vi "Generate a random block.vi"() -> (1 "Block Array":u8[][](array[numeric]))   [LabVIEW 2019]
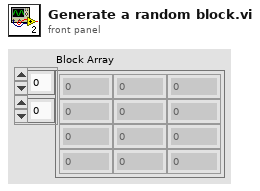
[diagram p1: front panel]
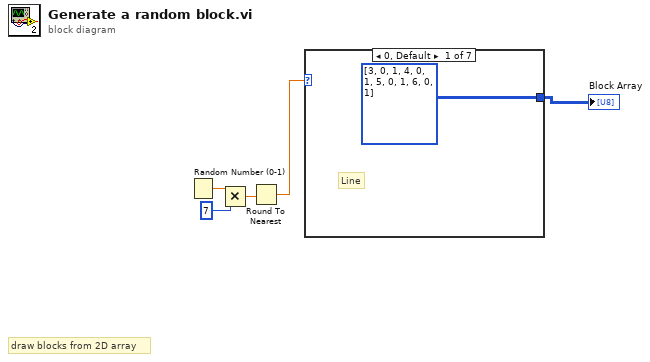
[diagram p0: block diagram]
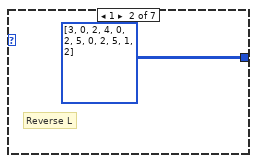
[diagram p2: hidden frame]
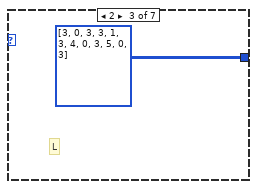
[diagram p3: hidden frame]
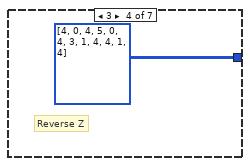
[diagram p4: hidden frame]
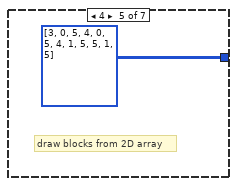
[diagram p5: hidden frame]
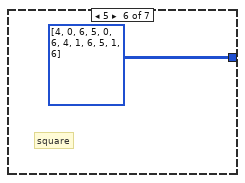
[diagram p6: hidden frame]
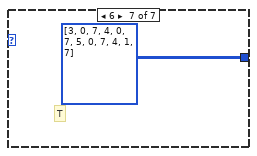
[diagram p7: hidden frame]
diagram:
  # "draw blocks from 2D array"
  n1 = Random Number (0-1)() -> (number: 0 to 1=w2:dbl)
  n2 = Multiply(x=w2, y=7) -> (x*y=w4:dbl)
  n3 = Round To Nearest(number=w4) -> (nearest integer value=w5:dbl)
  n4 = case shown="0, Default" w5 {
    tunnel: [u8[][] [[3, 0, 1], [4, 0, 1], [5, 0, 1], [6, 0, 1]] u8[][] [[3, 0, 2], [4, 0, 2], [5, 0, 2], [5, 1, 2]] u8[][] [[3, 0, 3], [3, 1, 3], [4, 0, 3], [5, 0, 3]] u8[][] [[4, 0, 4], [5, 0, 4], [3, 1, 4], [4, 1, 4]] u8[][] [[3, 0, 5], [4, 0, 5], [4, 1, 5], [5, 1, 5]] u8[][] [[4, 0, 6], [5, 0, 6], [4, 1, 6], [5, 1, 6]] u8[][] [[3, 0, 7], [4, 0, 7], [5, 0, 7], [4, 1, 7]]] -> w1
    frame 0, Default {
      # "Line"
    }
    frame 1 {
      # "Reverse L"
    }
    frame 2 {
      # "L"
    }
    frame 3 {
      # "Reverse Z"
    }
    frame 4 {
      # "draw blocks from 2D array"
    }
    frame 5 {
      # "square"
    }
    frame 6 {
      # "T"
    }
  }
  "Block Array" <- w1
